vi "Virtual Instr From JSON.vi"(8 "error in":errorcluster, 11 "Virt Instr JSON Config":path) -> (0 "error out":errorcluster, 3 "Virtual Instrument Base":refnum<class "Virtual Instrument Base.lvclass">)   [LabVIEW 2023]
uses:
  <vilib>/JDP Science/JSONtext/Config Files/Config File.lvclass
  <vilib>/ErrorRing/Error Ring.xnode
  <vilib>/Utility/error.llb/Error Cluster From Error Code.vi
  387fe87d-14ee-491f-8592-fd49c9380567.vi
  Virtual Instrument Base/Virtual Instrument Base.lvclass
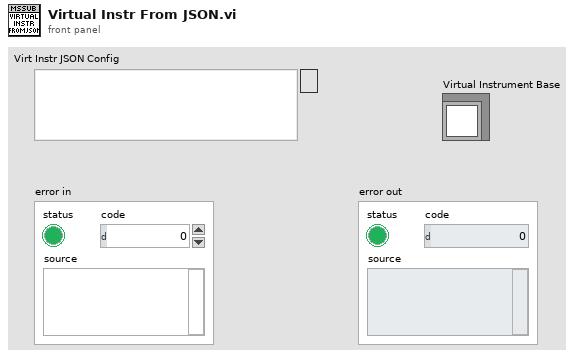
[diagram p1: front panel]
types:
  T1 = cluster{"Target Ident":string, "Action Data":variant, "Class":string}
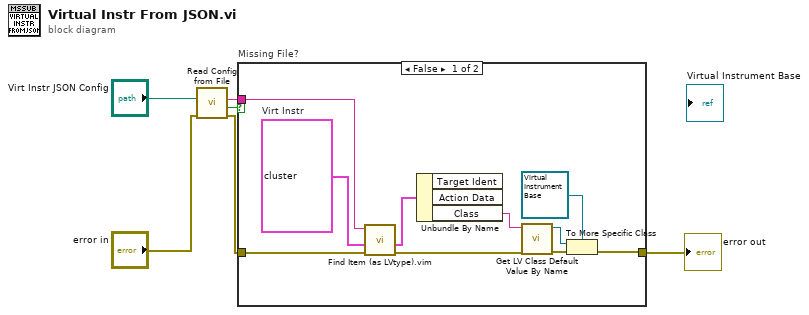
[diagram p0: block diagram]
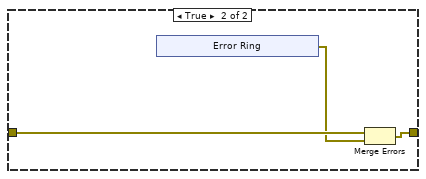
[diagram p2: hidden frame]
diagram:
  n1 = call <vilib>:"Read Config from File.vi"("error in (no error)"="error in", "config file path"="Virt Instr JSON Config") -> ("error out"=w3:errorcluster, "Template Used (file missing or corrupted)"=w4:bool, "<JSON>Config"=w1:string)  [unwired: 6 in, 1 out]
  n2 = case "Missing File?" shown="False" w4 {
    tunnel: w3 -> [w16 w19]
    tunnel: [w7 w17] -> w2
    tunnel: w1 -> [w15 _]
    frame False {
      w14 = T1 {"Target Ident"="", "Action Data"=variant, "Class"=""}  # Virt Instr
      n3 = call "Find Item (as LVtype).vim"("error in (no error)"=w16, "Data Type and Default Value"=w14, "JSON"=w15) -> ("error out"=w12:errorcluster, "Data"=w13:T1)  [unwired: 5 in, 2 out]
      n4 = Unbundle By Name(w13) -> ("Class"=w11:string)  [unwired: 2 out]
      n5 = call <vilib>:"Get LV Class Default Value By Name.vi"("error in (no error)"=w12, "class name"=w11) -> ("error out"=w10:errorcluster, "object"=w9:refnum<class>)  [unwired: 8 in]
      n6 = To More Specific Class(target class=refnum<class "Virtual Instrument Base.lvclass"> refnum ("Virtual Instrument Base.lvclass 2"), reference=w9, error in=w10) -> (error out=w7:errorcluster)  [unwired: 1 out]
    }
    frame True {
      n7 = xnode "Error Ring"() -> ("error out"=w18:errorcluster)
      n8 = Merge Errors(w19, w18) -> (w17:errorcluster)
    }
  }
  "error out" <- w2
